vi "Main_Example.vi"() -> ()   [LabVIEW 2015]
uses:
  controls/exampleControlCluster.ctl
  controls/clusterMain.ctl
  iniFileU32Type.vi
  iniFileBooleanType.vi
  iniFileStringType.vi
  <vilib>/Utility/config.llb/NI_LVConfig.lvlib
panel:
  out "error out":errorcluster
  out "Flags":T1
  in  "cfg":path
  # "Developed by Ezequiel Gonzalez\nPlastilinapps.com 2015"
  # "DIOinterface"
  # "UILang"
  # "DatabaseCon"
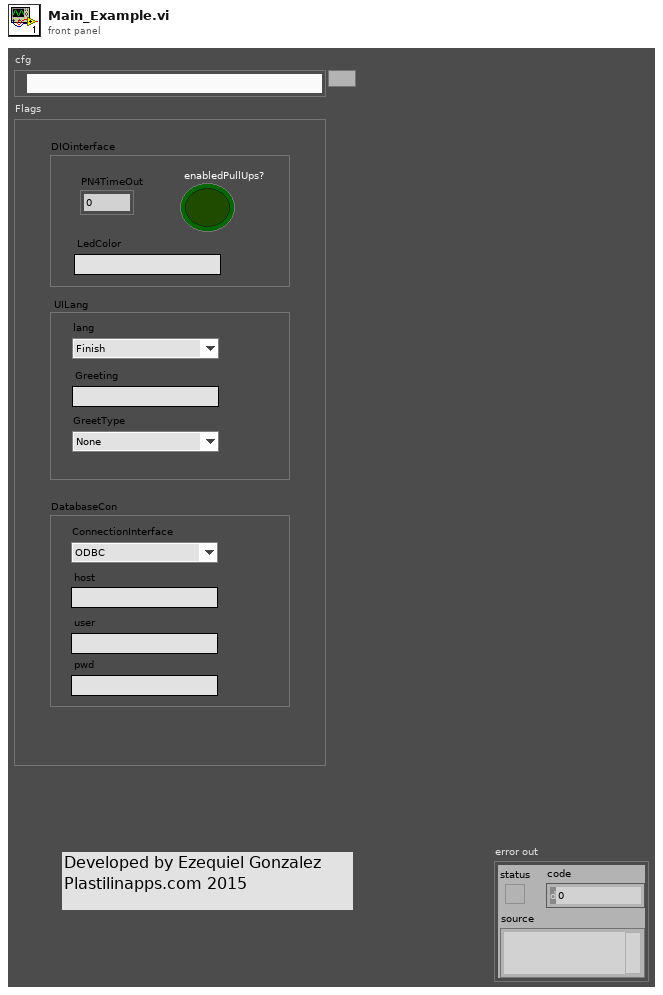
[diagram p1: front panel]
types:
  T1 = typedef "exampleControlCluster.ctl" = cluster{"PN4TimeOut":i32, "enabledPullUps?":T2, "LedColor":string, "lang":enum32{"Finish", "English", "Spanish", "French", "Japanese", "German", "Hebrew"}, "Greeting":string, "GreetType":enum32{"None", "PopUp", "Modal"}, "ConnectionInterface":enum32{"ODBC", "ADO", "JDBC"}, "host":string, "user":string, "pwd":string}
  T2 = typedef "clusterMain.ctl" = bool
  T3 = enum32{"Finish", "English", "Spanish", "French", "Japanese", "German", "Hebrew"}
  T4 = typedef "NI_LVConfig.lvlib/Config Data RefNum.ctl" = refnum<k1>
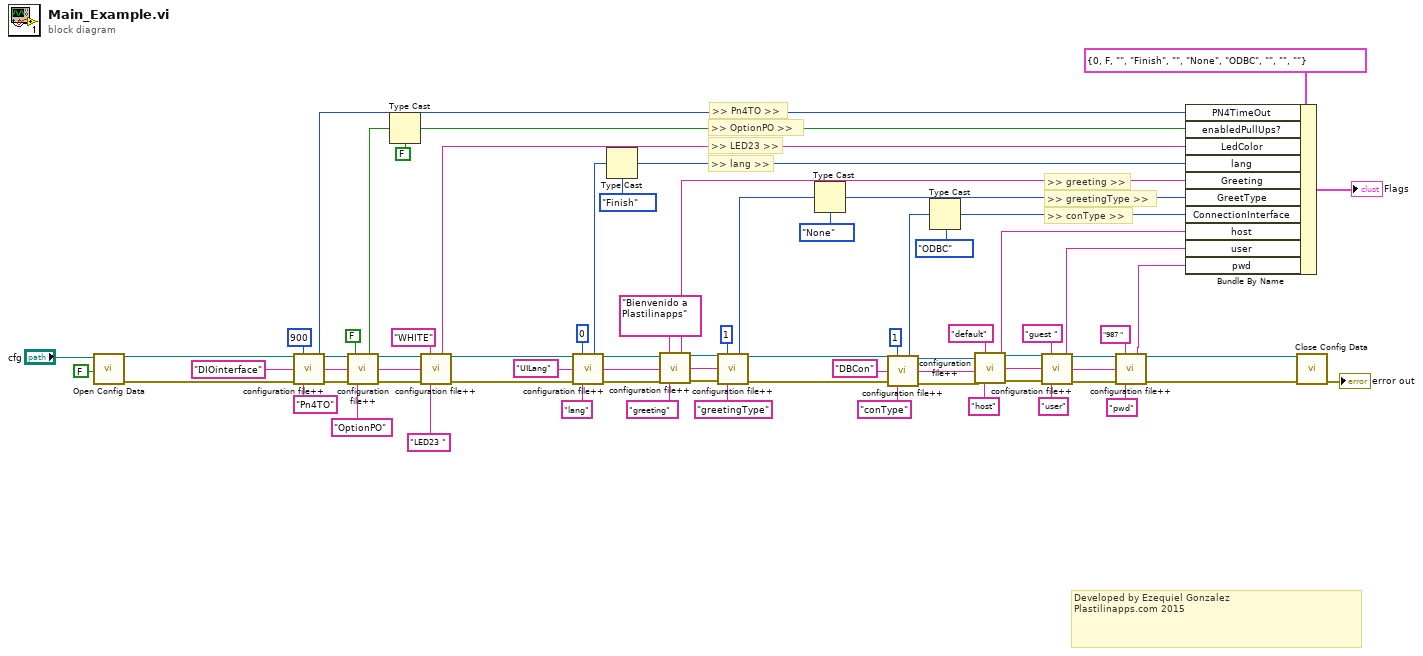
[diagram p0: block diagram]
diagram:
  # "Developed by Ezequiel Gonzalez\nPlastilinapps.com 2015"
  # ">> conType >>"
  # ">> greetingType >>"
  # ">> greeting >>"
  # ">> lang >>"
  # ">> LED23 >>"
  # ">> OptionPO >>"
  # ">> Pn4TO >>"
  n1 = call <vilib>:"Open Config Data.vi"("create file if necessary (T)"=FALSE, "configuration file path"="cfg") -> ("error out"=w74:errorcluster, "refnum"=w75:T4)  [unwired: 7 in, 1 out]
  n2 = call-poly "configuration file++.vi"("refnum"=w75, "default value"=u32 900, "section"="DIOinterface", "error in (no error)"=w74, "key"="Pn4TO") -> ("value"=w63:u32, "refnum out"=w69:T4, "section dup"=w70:string, "error out"=w68:errorcluster)  [unwired: 6 in, 1 out]
  n3 = call-poly "configuration file++.vi"("refnum"=w69, "default value"=FALSE, "section"=w70, "error in (no error)"=w68, "key"="OptionPO") -> ("value"=w37:bool, "refnum out"=w61:T4, "section dup"=w59:string, "error out"=w60:errorcluster)  [unwired: 6 in, 1 out]
  n4 = Type Cast(type=T2 FALSE ("enabledPullUps?"), x=w37) -> (*(type *) &x=w36:T2)
  n5 = call-poly "configuration file++.vi"("refnum"=w61, "default value"="WHITE", "section"=w59, "error in (no error)"=w60, "key"="LED23 ") -> ("value"=w56:string, "refnum out"=w54:T4, "error out"=w53:errorcluster)  [unwired: 6 in, 2 out]
  n6 = call-poly "configuration file++.vi"("refnum"=w54, "default value"=u32 0, "section"="UILang", "error in (no error)"=w53, "key"="lang") -> ("value"=w3:u32, "refnum out"=w50:T4, "section dup"=w48:string, "error out"=w49:errorcluster)  [unwired: 6 in, 1 out]
  n7 = Type Cast(type=T3."Finish" ("lang"), x=w3) -> (*(type *) &x=w1:T3)
  n8 = call-poly "configuration file++.vi"("refnum"=w50, "default value"="Bienvenido a Plastilinapps", "section"=w48, "error in (no error)"=w49, "key"="greeting") -> ("value"=w39:string, "refnum out"=w45:T4, "section dup"=w44:string, "error out"=w43:errorcluster)  [unwired: 6 in, 1 out]
  n9 = call-poly "configuration file++.vi"("refnum"=w45, "default value"=u32 1, "section"=w44, "error in (no error)"=w43, "key"="greetingType") -> ("value"=w6:u32, "refnum out"=w35:T4, "error out"=w34:errorcluster)  [unwired: 6 in, 2 out]
  n10 = Type Cast(type=enum32{"None", "PopUp", "Modal"}."None" ("GreetType"), x=w6) -> (*(type *) &x=w4:enum32{"None", "PopUp", "Modal"})
  n11 = call-poly "configuration file++.vi"("refnum"=w35, "default value"=u32 1, "section"="DBCon", "error in (no error)"=w34, "key"="conType") -> ("value"=w9:u32, "refnum out"=w30:T4, "section dup"=w29:string, "error out"=w28:errorcluster)  [unwired: 6 in, 1 out]
  n12 = Type Cast(type=enum32{"ODBC", "ADO", "JDBC"}."ODBC" ("ConnectionInterface"), x=w9) -> (*(type *) &x=w7:enum32{"ODBC", "ADO", "JDBC"})
  n13 = call-poly "configuration file++.vi"("refnum"=w30, "default value"="default", "section"=w29, "error in (no error)"=w28, "key"="host") -> ("value"=w26:string, "refnum out"=w24:T4, "section dup"=w23:string, "error out"=w22:errorcluster)  [unwired: 6 in, 1 out]
  n14 = call-poly "configuration file++.vi"("refnum"=w24, "default value"="guest ", "section"=w23, "error in (no error)"=w22, "key"="user") -> ("value"=w20:string, "refnum out"=w18:T4, "section dup"=w17:string, "error out"=w16:errorcluster)  [unwired: 6 in, 1 out]
  n15 = call-poly "configuration file++.vi"("refnum"=w18, "default value"="987 ", "section"=w17, "error in (no error)"=w16, "key"="pwd") -> ("value"=w13:string, "refnum out"=w12:T4, "error out"=w11:errorcluster)  [unwired: 6 in, 2 out]
  n16 = Bundle By Name(cluster=T1 {"PN4TimeOut"=0, "enabledPullUps?"=FALSE, "LedColor"="", "lang"=enum."Finish", "Greeting"="", "GreetType"=enum."None", "ConnectionInterface"=enum."ODBC", "host"="", "user"="", "pwd"=""} ("Cluster"), "PN4TimeOut"=w63, "enabledPullUps?"=w36, "LedColor"=w56, "lang"=w1, "Greeting"=w39, "GreetType"=w4, "ConnectionInterface"=w7, "host"=w26, "user"=w20, "pwd"=w13) -> (→"Flags":T1)
  n17 = call <vilib>:"Close Config Data.vi"("error in (no error)"=w11, "refnum"=w12) -> ("error out"=→"error out":errorcluster)  [unwired: 8 in, 1 out]
